vi "DataToOrigineGen.vi"(4 "UnitésDon":string[](array[string])=["(V)", "(°)"], 5 "Scan Names":string[](array[string]), 6 "Add X":bool caption="Add X Data", 7 "XName":string[](array[string]), 8 "error in":errorcluster, 9 "AllYData":dbl[][](array[numeric]), 10 "XData":dbl[][](array[numeric]), 11 "Origin.IOApp In":refnum<k7>) -> (0 "error IO":errorcluster, 3 "Origin.IOApp Out":refnum<k7>)   [LabVIEW 2010]
uses:
  <vilib>/regexp/Match Regular Expression.xnode
panel:
  out "Worksheet":refnum<k7>
  # "X Name format : \"Paramètre (unités)\""
  # "Le nom qui va dans l'espace \"comment\" \nex: \"pos(mm) Crb1\" donne \"pos Crb 1\""
  # ":Va dans l'entête de colonne"
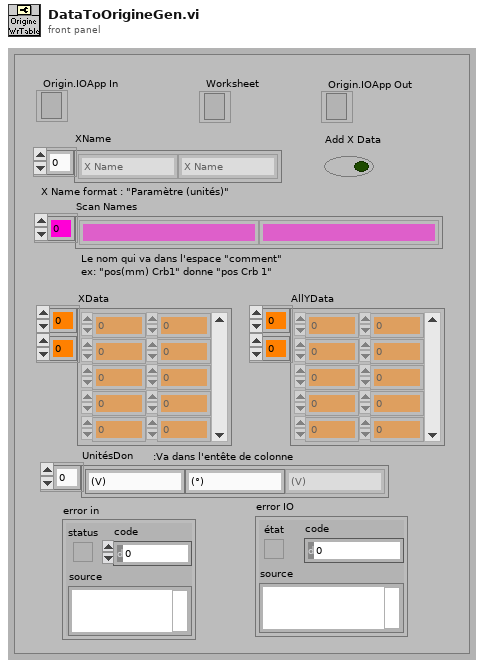
[diagram p1: front panel]
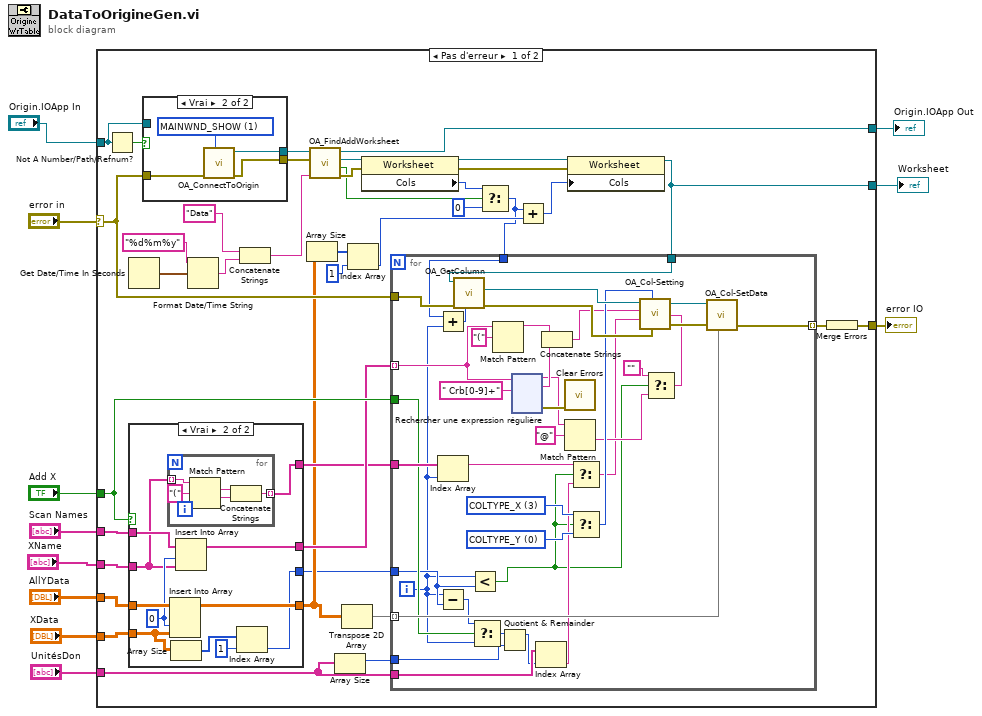
[diagram p0: block diagram]
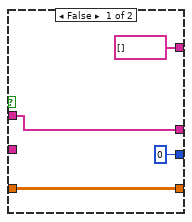
[diagram p2: hidden frame]
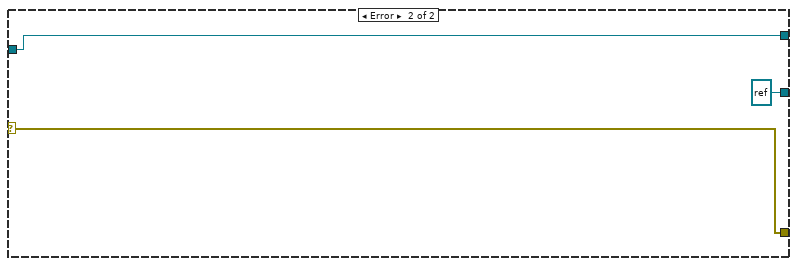
[diagram p4: hidden frame]
diagram:
  n1 = case shown="Pas d'erreur" "error in" {
    selector: "error in" -> [w47 w227]
    tunnel: "AllYData" -> [w30 _]
    tunnel: "Scan Names" -> [w29 _]
    tunnel: "Origin.IOApp In" -> [w21 w226]
    tunnel: "Add X" -> [w31 _]
    tunnel: "XName" -> [w27 _]
    tunnel: "XData" -> [w34 _]
    tunnel: [w32 w227] -> w5
    tunnel: [w22 w226] -> w4
    tunnel: [w17 refnum<k7> refnum ("Origin.Worksheet")] -> w3
    tunnel: "UnitésDon" -> [w14 _]
    frame No Error {
      n2 = Not A Number/Path/Refnum?(number/path/refnum=w21) -> (NaN/Path/Refnum?=w38:bool)
      n3 = Get Date/Time In Seconds() -> (seconds since 1Jan1904=w26:timestamp)
      n4 = case shown="Vrai" w31 {
        tunnel: w30 -> [w53 w64]
        tunnel: w34 -> [_ w59]
        tunnel: [w53 w63] -> w13
        tunnel: w29 -> [w52 w56]
        tunnel: [w52 w62] -> w28
        tunnel: w27 -> [_ w55]
        tunnel: [string[] [] w60] -> w15
        tunnel: [0 w54] -> w12
        frame False {
        }
        frame True {
          w61 = 0 ("indice désactivé (col)")
          n5 = for {
            tunnel: [w66] -> w60 mode=indexing
            tunnel: w55 -> [w65] mode=indexing
            n6 = Match Pattern(string=w65, regular expression="(" ("expression régulière")) -> (match substring=w68:string, after substring=w69:string)  [unwired: 1 in, 2 out]
            n7 = Concatenate Strings(w68, w69) -> (w66:string)
          }
          n8 = Insert Into Array(array=w64, index (col)=w61, new element=w59) -> (w63:dbl[][])  [unwired: 1 in]
          n9 = Array Size(array=w59) -> (size(s)=w58:i32[])
          n10 = Insert Into Array(array=w56, index=w61, new element=w55) -> (w62:string[])
          n11 = Index Array(array=w58, index=1) -> (element=w54:i32)
        }
      }
      n12 = case shown="Vrai" w38 {
        tunnel: [w70 w74] -> w49
        tunnel: [w71 w73] -> w48
        tunnel: w47 -> [w71 w72]
        tunnel: w21 -> [w70 _]
        frame False {
        }
        frame True {
          w75 = 1 items=["MAINWND_HIDE"=0, "MAINWND_SHOW"=1, "MAINWND_SHOWMINIMIZED"=2, "MAINWND_SHOWMAXIMIZED"=3, "MAINWND_SHOW_BRING_TO_FRONT"=100] ("Visible")
          n13 = call <userlib>:"OA_ConnectToOrigin.vi"("Visible"=w75, "error in (no error)"=w72) -> ("error out"=w73:errorcluster, "Origin.IOApplication"=w74:refnum<k7>)  [unwired: 6 in]
        }
      }
      n14 = Format Date/Time String(time format string (%c)="%d%m%y" ("chaîne de format de l'heure (%c)"), seconds (now)=w26) -> (date/time string=w20:string)  [unwired: 1 in]
      n15 = Concatenate Strings("Data" ("chaîne"), w20) -> (w18:string)
      n16 = Array Size(array=w13) -> (size(s)=w42:i32[])
      n17 = call <userlib>:"OA_FindAddWorksheet.vi"("Worksheet Name"=w18, "error in (no error)"=w48, "Origin.IOApplication"=w49) -> ("error out"=w45:errorcluster, "Found"=w37:bool, "Origin.Worksheet"=w46:refnum<k7>, "Origin.IOApplication"=w22:refnum<k7>)  [unwired: 2 in]
      n18 = Array Size(array=w14) -> (size(s)=w16:i32)
      n19 = Transpose 2D Array(2D array=w13) -> (transposed array=w24:dbl[][])
      n20 = Index Array(array=w42, index=1 ("indice")) -> (element=w39:i32)
      n21 = property class="Worksheet"(reference=w46, error in=w45) -> (reference out=w44:refnum<k7>, error out=w43:errorcluster, "Cols"=w36:i32)
      n22 = Select(t=w36, s=w37, f=0 ("cas faux")) -> (s? t:f=w23:i32)
      n23 = Add(x=w23, y=w39) -> (x+y=w40:i32)
      n24 = property class="Worksheet"(reference=w44, error in=w43, "Cols"=w40) -> (reference out=w17:refnum<k7>)  [unwired: 1 out]
      n25 = for {
        tunnel: w47 -> [w113]
        tunnel: w17 -> [w112]
        tunnel: w23 -> [w111]
        tunnel: w31 -> [w83]
        tunnel: w24 -> [w100] mode=indexing
        tunnel: [w99] -> w33 mode=indexing
        tunnel: w28 -> [w92] mode=indexing
        tunnel: w14 -> [w87]
        tunnel: w16 -> [w88]
        tunnel: w15 -> [w84]
        tunnel: w12 -> [w78]
        i -> [w77]
        w107 = 0 items=["COLTYPE_NO_CHANGE"=-1, "COLTYPE_Y"=0, "COLTYPE_NONE"=1, "COLTYPE_ERROR"=2, "COLTYPE_X"=3, "COLTYPE_LABEL"=4, "COLTYPE_Z"=5, "COLTYPE_X_ERROR"=6, "COLTYPE_GROUP"=7, "COLTYPE_SUBJECT"=8] ("Type")
        w105 = 3 items=["COLTYPE_NO_CHANGE"=-1, "COLTYPE_Y"=0, "COLTYPE_NONE"=1, "COLTYPE_ERROR"=2, "COLTYPE_X"=3, "COLTYPE_LABEL"=4, "COLTYPE_Z"=5, "COLTYPE_X_ERROR"=6, "COLTYPE_GROUP"=7, "COLTYPE_SUBJECT"=8] ("Type")
        n26 = Add(x=w111, y=w77) -> (x+y=w110:i32)
        n27 = Index Array(array=w84, index=w77) -> (element=w79:string)
        n28 = Subtract(x=w77, y=w78) -> (x-y=w76:i32)
        n29 = call <userlib>:"OA_GetColumn.vi"("Column Name/Index"=w110, "error in (no error)"=w113, "Origin.Worksheet"=w112) -> ("error out"=w109:errorcluster, "Origin.Column"=w108:refnum<k7>)  [unwired: 6 in, 1 out]
        n30 = Less?(x=w77, y=w78) -> (x < y?=w80:bool)
        n31 = Select(t=w76, s=w83, f=w77) -> (s? t:f=w81:i32)
        n32 = Match Pattern(string=w92, regular expression="(" ("expression régulière")) -> (before substring=w103:string)  [unwired: 1 in, 3 out]
        n33 = Quotient & Remainder(x=w81, y=w88) -> (x-y*floor(x/y)=w82:i32)  [unwired: 1 out]
        n34 = xnode "Rechercher une expression régulière"("chaîne en entrée"=w92, "expression régulière"=" Crb[0-9]+") -> ("avant la correspondance"=w90:string, "toute l'expression"=w94:string, "sortie d'erreur"=w93:errorcluster)  [unwired: 4 in, 2 out]
        n35 = Index Array(array=w87, index=w82) -> (element=w86:string)
        n36 = Concatenate Strings(w103, w94) -> (w98:string)
        n37 = call <vilib>:"Clear Errors.vi"("error in (no error)"=w93) -> ()  [unwired: 6 in, 1 out]
        n38 = Match Pattern(string=w90, regular expression="@") -> (after substring=w89:string)  [unwired: 1 in, 3 out]
        n39 = Select(t=w79, s=w80, f=w86) -> (s? t:f=w85:string)
        n40 = Select(t=w105, s=w80, f=w107) -> (s? t:f=w106:i32)
        n41 = Select(t="", s=w80, f=w89) -> (s? t:f=w95:string)
        n42 = call <userlib>:"OA_Col-Setting.vi"("Origin.Column"=w108, "Type"=w106, "LongName"=w98, "Units"=w85, "error in (no error)"=w109, "Comments"=w95) -> ("Origin.Column Out"=w101:refnum<k7>, "error out"=w102:errorcluster)  [unwired: 1 in]
        n43 = call <userlib>:"OA_Col-SetData.vi"("Origin.Column"=w101, "error in (no error)"=w102, "data"=w100) -> ("error out"=w99:errorcluster)  [unwired: 4 in, 2 out]
      }
      n44 = Merge Errors(w33) -> (w32:errorcluster)
    }
    frame Error {
    }
  }
  "error IO" <- w5
  "Origin.IOApp Out" <- w4
  "Worksheet" <- w3
